vi "finish.vi"(8 "error in (no error)":errorcluster, 11 "Pneumatics in":refnum<class "Pneumatics.lvclass">) -> (0 "error out":errorcluster, 3 "Pneumatics out":refnum<class "Pneumatics.lvclass">)   [LabVIEW 2018, in "Pneumatics control.lvlib" / "Pneumatics.lvclass"]
doc: "This closes the solonoids for the Pnuematics class."
uses:
  Pneumatics.lvclass
  Pneumatics.lvclass/Pneumatics.ctl
  <vilib>/Rock Robotics/WPI/Utilities/WPI_GetSetVariantRefNum.vi
  Solenoids/Solenoids.lvclass
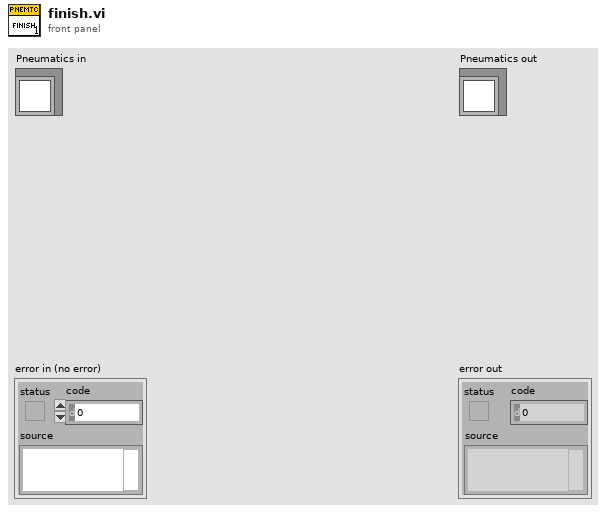
[diagram p1: front panel]
types:
  T1 = typedef "Pneumatics control.lvlib/Pneumatics.lvclass/Solenoids.ctl" = cluster{"DriveShift":refnum<class "Solenoids.lvclass">, "ArmLock":refnum<class "Solenoids.lvclass">, "HatchArm":refnum<class "Solenoids.lvclass">, "HatchGrabber":refnum<class "Solenoids.lvclass">}
  T2 = typedef "WPI_CompressorDevRef.ctl" = cluster{"DevStatus":errorcluster, "Pneumatics Control Module":u8}
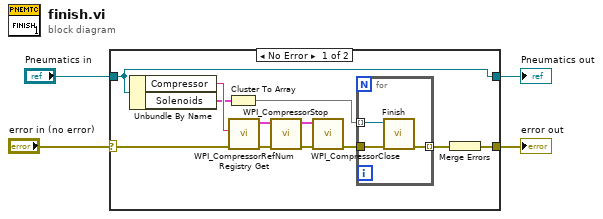
[diagram p0: block diagram]
diagram:
  n1 = case shown="No Error" "error in (no error)" {
    selector: "error in (no error)" -> [w7 w21]
    tunnel: [w5 w21] -> w3
    tunnel: [w12 w20] -> w1
    tunnel: "Pneumatics in" -> [w12 w20]
    frame No Error {
      n2 = Unbundle By Name(w12) -> ("Compressor"=w11:string, "Solenoids"=w10:T1)
      n3 = Cluster To Array(cluster=w10) -> (array=w9:refnum<class "Solenoids.lvclass">[])
      n4 = call <vilib>:"WPI_CompressorRefNum Registry Get.vi"("error in (no error)"=w7, "refnum name"=w11) -> ("error out"=w13:errorcluster, "CompressorDevRef"=w14:T2)  [unwired: 8 in]
      n5 = call <vilib>:"WPI_CompressorStop.vi"("error in (no error)"=w13, "CompressorDevRef"=w14) -> ("error out"=w15:errorcluster, "CompressorDevRef"=w16:T2)  [unwired: 8 in]
      n6 = call <vilib>:"WPI_CompressorClose.vi"("error in (no error)"=w15, "CompressorDevRef"=w16) -> ("error out"=w8:errorcluster)  [unwired: 9 in]
      n7 = for {
        tunnel: w9 -> [w19] mode=indexing
        tunnel: w8 -> [w18]
        tunnel: [w17] -> w6 mode=indexing
        n8 = call-dynamic "Finish.vi"("error in (no error)"=w18, "Solenoids in"=w19) -> ("error out"=w17:errorcluster)  [unwired: 8 in, 1 out]
      }
      n9 = Merge Errors(w6) -> (w5:errorcluster)
    }
    frame Error {
    }
  }
  "error out" <- w3
  "Pneumatics out" <- w1
